vi "Operation flags DSP402.vi"(6 "Bit 6":T1 items=["---", "OFF", "ON"], 7 "Halt":T1 items=["---", "OFF", "ON"], 8 "error in (no error)":errorcluster, 9 "Bit 5":T1 items=["---", "OFF", "ON"], 10 "Bit 4":T1 items=["---", "OFF", "ON"], 11 "DSP402 in":refnum<class "DSP402.lvclass">) -> (0 "error out":errorcluster, 3 "DSP402 out":refnum<class "DSP402.lvclass">)   [LabVIEW 2026, in "canopen_.lvlib" / "DSP402.lvclass"]
uses:
  DSP402.lvclass
  DSP402.lvclass/DSP402.ctl
  types/threestateFlag.ctl
  canopen_.lvlib
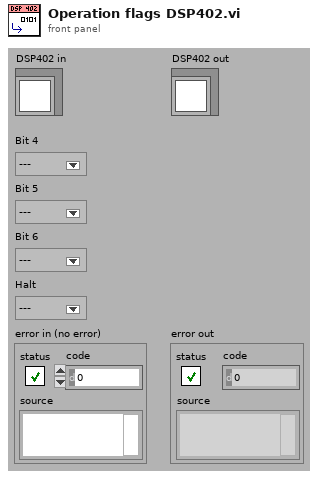
[diagram p1: front panel]
types:
  T1 = typedef "canopen_.lvlib/threestateFlag.ctl" = i8
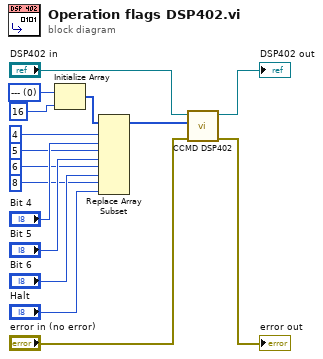
[diagram p0: block diagram]
diagram:
  w11 = T1 0 items=["---", "OFF", "ON"] ("New value")
  n1 = Initialize Array(w11, 16 ("dimension size")) -> (w10:T1[])
  n2 = Replace Array Subset(array=w10, new element #1="Bit 4", index #1=4 ("index"), new element #2="Bit 5", index #2=5 ("index"), new element #3="Bit 6", index #3=6 ("index"), new element #4="Halt", index #4=8 ("index")) -> (w1:T1[])
  n3 = call "CCMD DSP402.vi"("error in (no error)"="error in (no error)", "Mask"=w1, "DSP402 in"="DSP402 in") -> ("error out"=→"error out":errorcluster, "DSP402 out"=→"DSP402 out":refnum<class "DSP402.lvclass">)  [unwired: 3 out]
